vi "rad_FTP Check log folder size on Target.vi"(8 "error in (no error)":errorcluster, 10 "Target settings":T1={"Hostname"="", "Serial number"="", "Product name"="", "Product code"=0, "System status"="", "Credential type"=enum."None/Unlocked", "User added?"=FALSE, "Primary NIC"={"MAC address"="", "IP Address Request Mode"=2, "IP address"="", "Subnet mask"="", "Gateway"="", "DNS server"=""}} {"Primary NIC"."IP Address Request Mode" items=["Static"=1, "DHCP/Link-Local"=2, "Link-Local Only"=4, "DHCP Only"=8]}) -> (0 "error out":errorcluster)   [LabVIEW 2020]
uses:
  Targets/TypeDefs/rad_Target Information.ctl
  Targets/TypeDefs/rad_Target Network Settings.ctl
  <vilib>/FTP/NI_FTP.lvlib
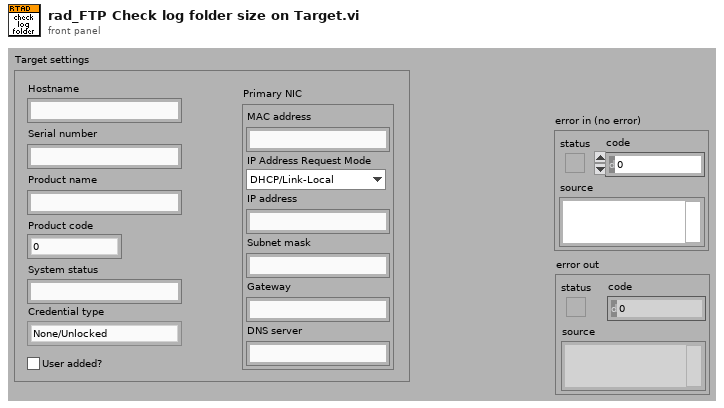
[diagram p1: front panel]
types:
  T1 = typedef "rad_Target Information.ctl" = cluster{"Hostname":string, "Serial number":string, "Product name":string, "Product code":i32, "System status":string, "Credential type":enum16{"None/Unlocked", "FTP Password", "NIAuth Credentials"}, "User added?":bool, "Primary NIC":T2}
  T2 = typedef "rad_Target Network Settings.ctl" = cluster{"MAC address":string, "IP Address Request Mode":i32, "IP address":string, "Subnet mask":string, "Gateway":string, "DNS server":string}
  T3 = typedef "NI_FTP.lvlib/FTP Session.ctl" = refnum<k5>
  T4 = typedef "NI_FTP.lvlib/FTP File Info.ctl" = cluster{"type":enum16{"unknown", "file", "dir", "link"}, "permissions":string, "owner":string, "group":string, "size":i32, "date":string, "name":string, "link name":string}
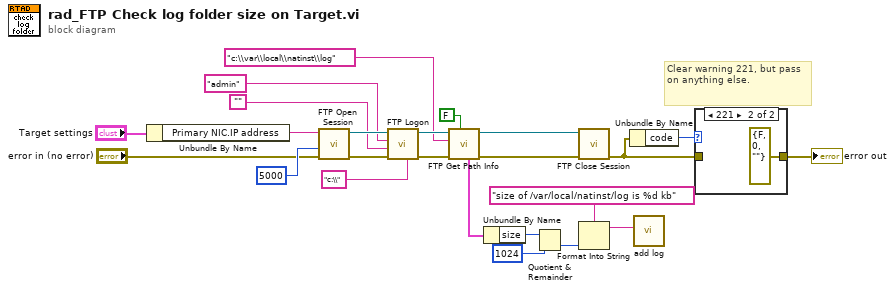
[diagram p0: block diagram]
diagram:
  # "Clear warning 221, but pass on anything else."
  n1 = Unbundle By Name("Target settings") -> ("Primary NIC.IP address"=w24:string)
  n2 = call <vilib>:"FTP Open Session.vi"("error in (no error)"="error in (no error)", "timeout ms (60000)"=5000, "address"=w24) -> ("error out"=w23:errorcluster, "ftp session"=w22:T3)  [unwired: 5 in, 2 out]
  n3 = call <vilib>:"FTP Logon.vi"("starting path"="c:\\" ("remote path"), "error in (no error)"=w23, "password"="", "user"="admin", "ftp session"=w22) -> ("error out"=w16:errorcluster, "ftp session out"=w15:T3)  [unwired: 3 in, 2 out]
  n4 = call <vilib>:"FTP Get Path Info.vi"("active (T)"=FALSE ("binary (F)"), "error in (no error)"=w16, "remote path"="c:\\var\\local\\natinst\\log", "ftp session"=w15) -> ("error out"=w9:errorcluster, "ftp session out"=w10:T3, "path info"=w11:T4)  [unwired: 3 in, 2 out]
  n5 = Unbundle By Name(w11) -> ("size"=w2:i32)
  n6 = Quotient & Remainder(x=w2, y=1024) -> (floor(x/y)=w3:i32)  [unwired: 1 out]
  n7 = call <vilib>:"FTP Close Session.vi"("error in (no error)"=w9, "ftp session"=w10) -> ("error out"=w7:errorcluster)  [unwired: 6 in, 3 out]
  n8 = Format Into String(format string="size of /var/local/natinst/log is %d kb" ("remote path"), w3) -> (resulting string=w5:string)  [unwired: 2 in, 1 out]
  n9 = Unbundle By Name(w7) -> ("code"=w8:i32)
  n10 = call "add log.vi"("text"=w5) -> ()  [unwired: 10 in, 1 out]
  n11 = case shown="221" w8 {
    tunnel: [w25 errorcluster {"status"=FALSE, "code"=0, "source"=""} ("error IO")] -> w6
    tunnel: w7 -> [w25 _]
    frame Default {
    }
    frame 221 {
    }
  }
  "error out" <- w6
